vi "Divide By Scalar.vi"(10 "x":sgl, 11 "A":refnum<class "Vector 2D.lvclass">) -> (3 "Ax":refnum<class "Vector 2D.lvclass">)   [LabVIEW 2021, in "Vector 2D.lvclass"]
uses:
  Vector 2D.lvclass
  Vector 2D.lvclass/Vector 2D.ctl
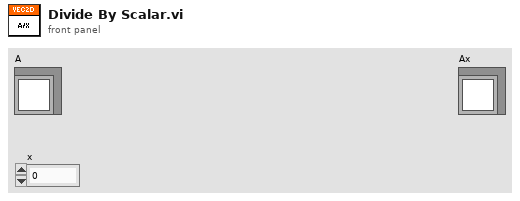
[diagram p1: front panel]
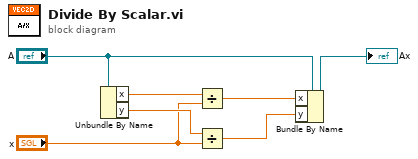
[diagram p0: block diagram]
diagram:
  n1 = Unbundle By Name("A") -> ("x"=w5:sgl, "y"=w4:sgl)
  n2 = Divide(x=w5, y="x") -> (x/y=w3:sgl)
  n3 = Divide(x=w4, y="x") -> (x/y=w2:sgl)
  n4 = Bundle By Name(cluster="A", "x"=w3, "y"=w2) -> (→"Ax":refnum<class "Vector 2D.lvclass">)
